vi "Tektronix TDS 3000 Series Auto Setup Waveform Acquire.vi"() -> ()   [LabVIEW 2010]
doc: "DESCRIPTION:\nThis VI shows how to acquire a waveform on the Tektronix TDS 3xxx Series using Auto Setup. \n\nINSTRUCTIONS:\n1. Pass a valid VISA session\n2. Enter the desired channel.\n3. The acquired waveform will be displayed in the graph."
uses:
  <instrlib>/Tektronix TDS 3000 Series/Tektronix TDS 3000 Series.lvlib
panel:
  in  "Channel (\"CH1\")":string(combo)="CH1"
  in  "VISA resource name":refnum<visa-resource-name>="GPIB0::1::INSTR"
  out "Waveform Graph":T1(graph)
  # "© 2003-2006, National Instruments, Corporation.  All Rights Reserved."
  # "For instructions,\nselect Show Context Help\nfrom the Help menu."
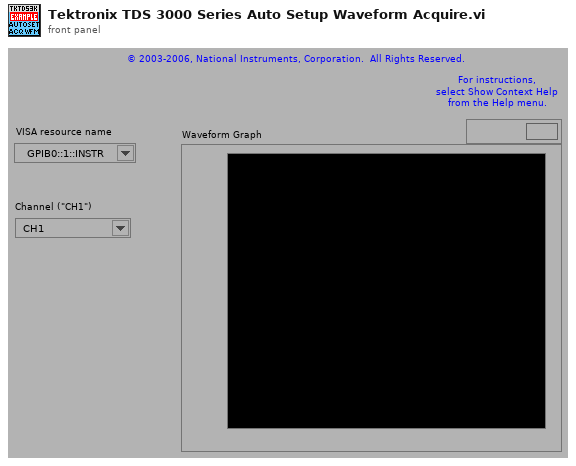
[diagram p1: front panel]
types:
  T1 = cluster{"Initial X":dbl, "X Increment":dbl, "Waveform Array":dbl[]}
  T2 = cluster{"Baud Rate (9600)":u32, "Flow Control (RTS/CTS)":u16, i32}
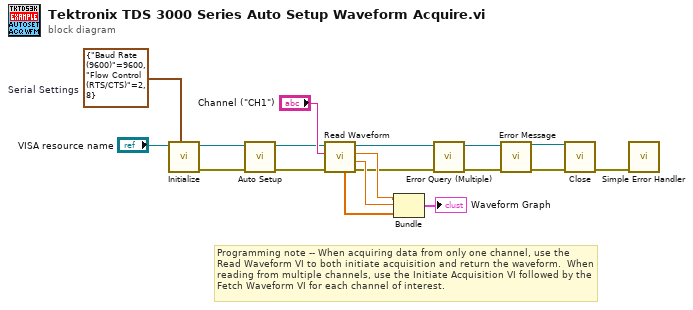
[diagram p0: block diagram]
diagram:
  w12 = T2 {"Baud Rate (9600)"=9600, "Flow Control (RTS/CTS)"=2, 8}  # Serial Settings
  # "Programming note -- When acquiring data from only one channel, use the Read Waveform VI to both initiate acquisition and return the waveform.  When reading from multiple channels, use the Initiate Acquisition VI followed by the Fetch Waveform VI for each channel of interest."
  n1 = call <instrlib>:"Initialize.vi"("Serial Settings"=w12, "VISA Resource Name"="VISA resource name") -> ("error out"=w1:errorcluster, "VISA Resource Name Out"=w2:refnum<visa-resource-name>)  [unwired: 8 in]
  n2 = call <instrlib>:"Auto Setup.vi"("error in (no error)"=w1, "VISA Resource Name"=w2) -> ("error out"=w3:errorcluster, "VISA Resource Name Out"=w4:refnum<visa-resource-name>)  [unwired: 8 in]
  n3 = call <instrlib>:"Read Waveform.vi"("error in (no error)"=w3, "Source (Channel 1)"="Channel (\"CH1\")", "VISA Resource Name"=w4) -> ("error out"=w10:errorcluster, "X Increment"=w16:dbl, "Initial X"=w15:dbl, "VISA Resource Name Out"=w11:refnum<visa-resource-name>, "Waveform Array"=w17:dbl[])  [unwired: 3 in, 1 out]
  n4 = Bundle("Initial X"=w15, "X Increment"=w16, "Waveform Array"=w17) -> (→"Waveform Graph":T1)  [unwired: 1 in]
  n5 = call <instrlib>:"Error Query (Multiple).vi"("error in (no error)"=w10, "VISA Resource Name"=w11) -> ("error out"=w8:errorcluster, "VISA Resource Name Out"=w9:refnum<visa-resource-name>)  [unwired: 6 in, 2 out]
  n6 = call <instrlib>:"Error Message.vi"("VISA Resource Name"=w9, "error in (no error)"=w8) -> ("VISA Resource Name Out"=w7:refnum<visa-resource-name>, "error out"=w6:errorcluster)  [unwired: 9 in, 3 out]
  n7 = call <instrlib>:"Close.vi"("error in (no error)"=w6, "VISA Resource Name"=w7) -> ("error out"=w5:errorcluster)  [unwired: 9 in]
  n8 = call <vilib>:"Simple Error Handler.vi"("error in (no error)"=w5) -> ()  [unwired: 4 in, 5 out]
